vi "ExtraFilter_2channel.vi"(5 "new coeffs":fxp<+/-,18,18>[](array[numeric]), 6 "reset":bool, 7 "new coeffs":bool, 8 "valid in":bool, 9 "enable filter":bool, 10 "new shift":i32, 11 "Data in":fxp<+/-,16,14>[](array[numeric])=[0.0, 0.0, 0.0, 0.0]) -> (0 "valid out":bool, 3 "Data out":fxp<+/-,16,14>[](array[numeric]))   [LabVIEW 2013]
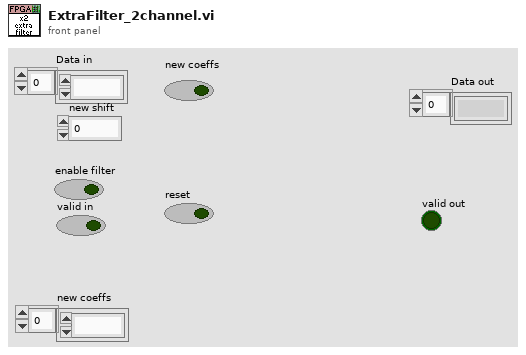
[diagram p1: front panel]
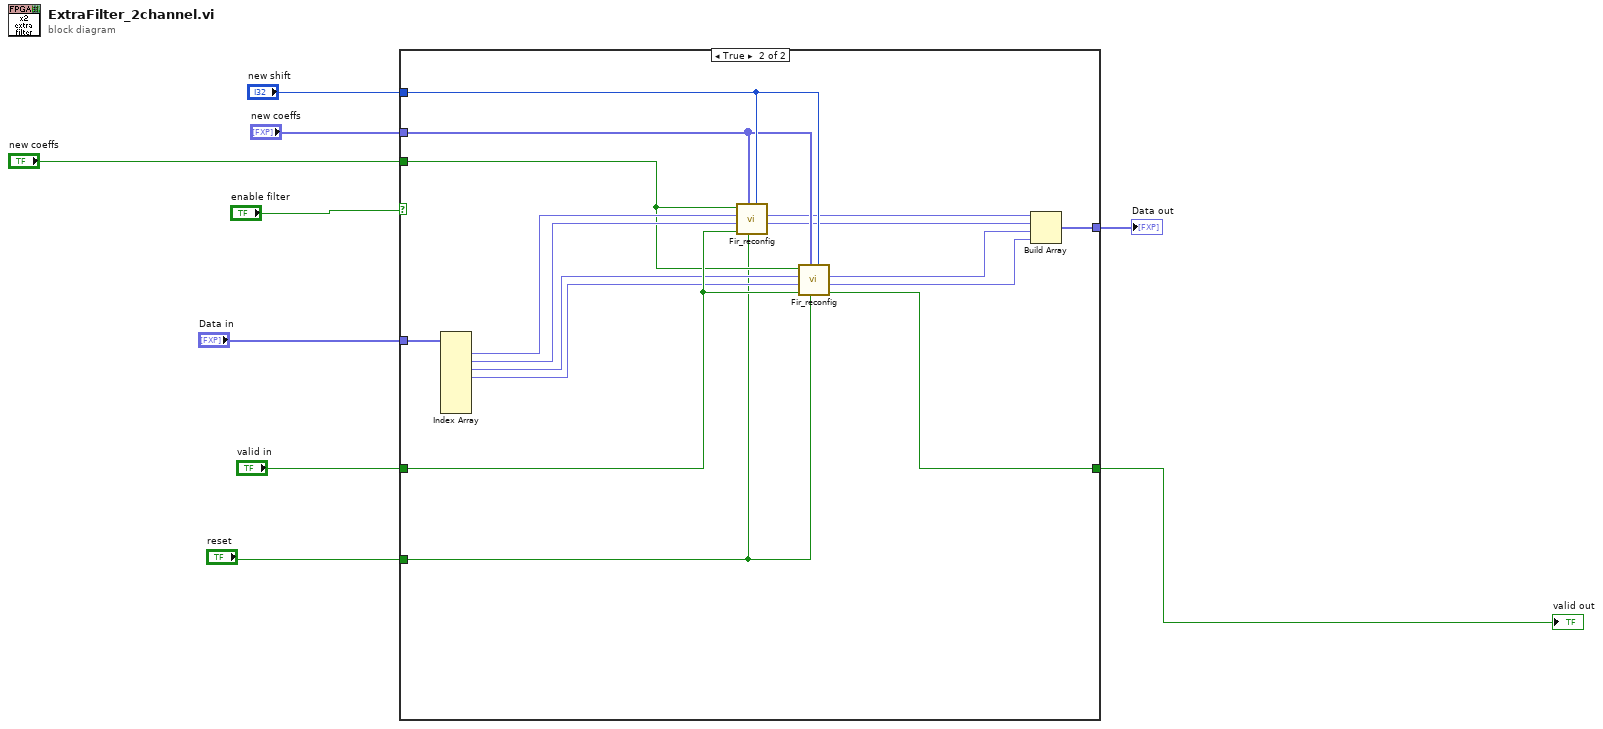
[diagram p0: block diagram]
diagram:
  n1 = case shown="True" "enable filter" {
    tunnel: "Data in" -> [w10 w27]
    tunnel: "valid in" -> [w11 w26]
    tunnel: "new coeffs" -> [_ w19]
    tunnel: [w11 w17] -> w2
    tunnel: "new shift" -> [_ w20]
    tunnel: "new coeffs" -> [_ w21]
    tunnel: "reset" -> [_ w18]
    tunnel: [w10 w12] -> w1
    frame False {
    }
    frame True {
      n2 = Index Array(array=w27) -> (element #1=w25:fxp<+/-,16,14>, element #2=w24:fxp<+/-,16,14>, element #3=w23:fxp<+/-,16,14>, element #4=w22:fxp<+/-,16,14>)  [unwired: 8 in, 4 out]
      n3 = call "Fir_reconfig.vi"("new shift"=w20, "reset"=w18, 7:"new coeffs"=w19, "valid in"=w26, "Q in"=w24, "I in"=w25, 11:"new coeffs"=w21) -> ("Q out"=w15:fxp<+/-,16,14>, "I out"=w16:fxp<+/-,16,14>)  [unwired: 1 in, 2 out]
      n4 = call "Fir_reconfig.vi"("new shift"=w20, "reset"=w18, 7:"new coeffs"=w19, "valid in"=w26, "Q in"=w22, "I in"=w23, 11:"new coeffs"=w21) -> ("valid out"=w17:bool, "Q out"=w13:fxp<+/-,16,14>, "I out"=w14:fxp<+/-,16,14>)  [unwired: 1 in, 1 out]
      n5 = Build Array(w16, w15, w14, w13) -> (w12:fxp<+/-,16,14>[])
    }
  }
  "valid out" <- w2
  "Data out" <- w1
